vi "open.vi"(8 "error in (no error)":errorcluster caption="错误输入（无错误）", 10 "index (row)":i8=75, 11 "6509_switch 输入":refnum<class "6509_switch.lvclass"> caption="DNL_LabVIEW Object in") -> (0 "error out":errorcluster caption="错误输出", 3 "6509_switch 输出":refnum<class "6509_switch.lvclass"> caption="DNL_LabVIEW Object out")   [LabVIEW 2011, in "6509_switch.lvclass"]
uses:
  6509_switch.lvclass
  6509_switch.lvclass/6509_switch.ctl
panel:
  in  "Lines 4":tag="Dev3/port0/line0:7, Dev3/port1/line0:7, Dev3/port2/line0:7, Dev3/port3/line0:7, Dev3/port4/line0:7, Dev3/port5/line0:7, Dev3/port6/line0:7, Dev3/port7/line0:7, Dev3/port8/line0:7, Dev3/port9/line0:7, Dev3/port10/line0:7, Dev3/port11/line0:7" caption="Lines"
  in  "Lines 2":tag="Dev2/port0/line0:7, Dev2/port1/line0:7, Dev2/port2/line0:7, Dev2/port3/line0:7, Dev2/port4/line0:7, Dev2/port5/line0:7, Dev2/port6/line0:7, Dev2/port7/line0:7, Dev2/port8/line0:7, Dev2/port9/line0:7, Dev2/port10/line0:7, Dev2/port11/line0:7" caption="Lines"
  in  "Lines":tag="Dev1/port0/line0:7, Dev1/port1/line0:7, Dev1/port2/line0:7, Dev1/port3/line0:7, Dev1/port4/line0:7, Dev1/port5/line0:7, Dev1/port6/line0:7, Dev1/port7/line0:7, Dev1/port8/line0:7, Dev1/port9/line0:7, Dev1/port10/line0:7, Dev1/port11/line0:7"
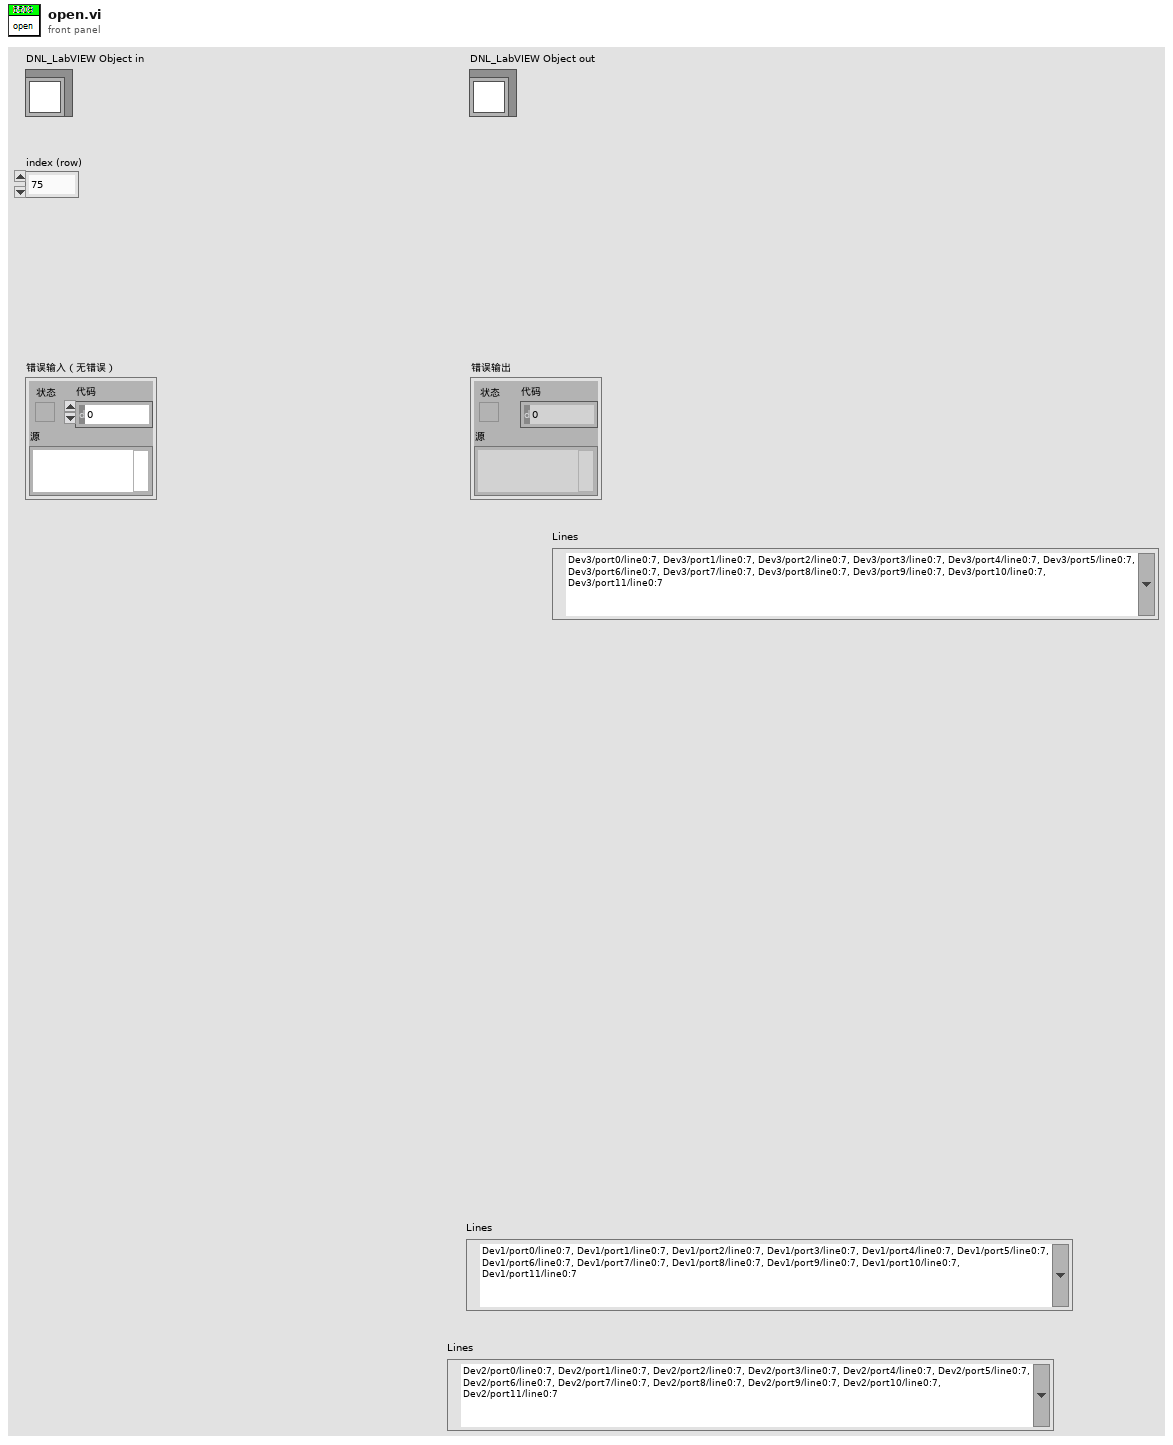
[diagram p1: front panel]
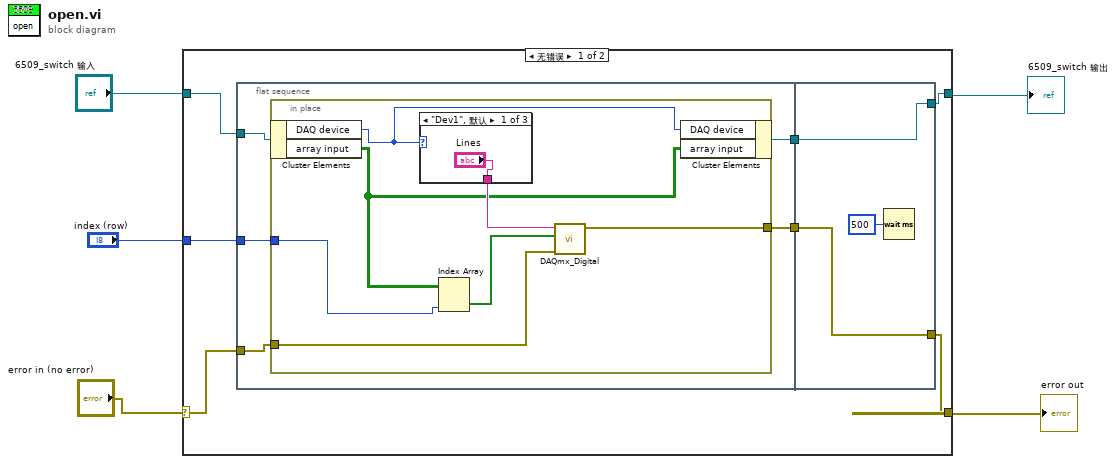
[diagram p0: block diagram]
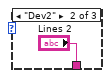
[diagram p2: hidden frame]
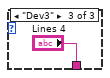
[diagram p3: hidden frame]
diagram:
  n1 = case shown="无错误" "error in (no error)" {
    selector: "error in (no error)" -> [w10 w31]
    tunnel: [w8 w31] -> w4
    tunnel: "6509_switch 输入" -> [w12 w32]
    tunnel: [w6 w32] -> w2
    tunnel: "index (row)" -> [w11 _]
    frame No Error {
      n2 = flat-sequence {
        tunnel: w12 -> [w17]
        tunnel: w11 -> [w16]
        tunnel: w10 -> [w15]
        tunnel: [w14] -> w9
        tunnel: [w13] -> w7
        tunnel: w9 -> [w29]
        tunnel: [w29] -> w8
        tunnel: w7 -> [w28]
        tunnel: [w28] -> w6
        frame #0 {
          n3 = in-place {
            in-place-border: w16 -> [w23]
            in-place-border: w15 -> [w21]
            in-place-border: [w20] -> w14
            n4 = in-place-cluster #1(w17) -> ("DAQ device"=w19:enum16{"Dev1", "Dev2", "Dev3"}, "array input"=w18:bool[][])
            n5 = case shown="\"Dev1\", 默认" w19 {
              tunnel: ["Lines" "Lines 2" "Lines 4"] -> w22
              frame "Dev1", Default {
              }
              frame "Dev2" {
              }
              frame "Dev3" {
              }
            }
            n6 = Index Array(array=w18, index (col)=w23) -> (element=w24:bool[])  [unwired: 1 in]
            n7 = call "DAQmx_Digital.vi"("Error in"=w21, "Data"=w24, "lines"=w22) -> ("Error out"=w20:errorcluster)  [unwired: 8 in]
            n8 = in-place-cluster #1("DAQ device"=w19, "array input"=w18) -> (w13:refnum<class "6509_switch.lvclass">)
          }
        }
        frame #1 {
          n9 = Wait (ms)(milliseconds to wait=u32 500 ("等待时间（毫秒）")) -> ()  [unwired: 1 out]
        }
      }
    }
    frame Error {
    }
  }
  "error out" <- w4
  "6509_switch 输出" <- w2
